vi "FdxCmdTxSAPCreatePortCvi.vi"(8 "error in":errorcluster, 9 "SapCreateIn":T1, 11 "InstrumentHandle":u32) -> (0 "error out":errorcluster, 1 "UdpHandle":u32, 3 "InstrumentHandle":u32)   [LabVIEW 2020, in "AIM664LV.lvlib"]
doc: "Creates an SAP type UDP port to transmit data from a specified UDP connectionless port. Default settings after creation of SAP port are:\n- UDP port enabled\n- Error injection: OFF\n- Skew (redundand mode only): 0 usec.\nTo change settings of the SAP port the function AiFdxCmdTxUDPControl can be used. This function can be used only, if transmitter is not running."
uses:
  AIM664LV.lvlib
  AFDX_LibraryAdmin/FdxGlobalDllPath.vi
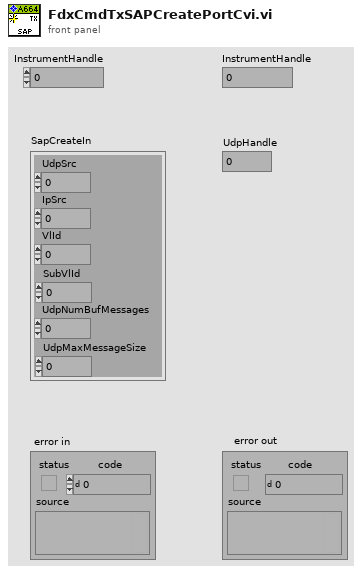
[diagram p1: front panel]
types:
  T1 = cluster{"UdpSrc":u32, "IpSrc":u32, "VlId":u32, "SubVlId":u32, "UdpNumBufMessages":u32, "UdpMaxMessageSize":u32}
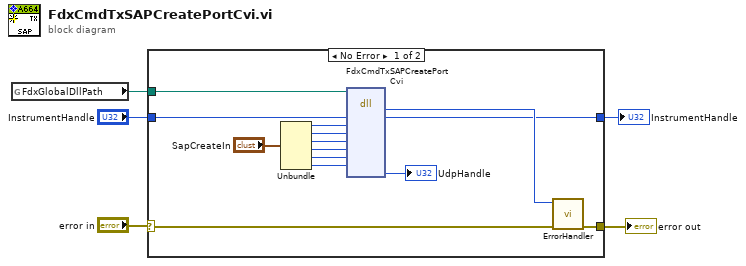
[diagram p0: block diagram]
diagram:
  n1 = global read "FdxGlobalDllPath.vi" "FdxGlobalDllPath"() -> (w3:path)
  n2 = case shown="No Error" "error in" {
    selector: "error in" -> [w18 w21]
    tunnel: [w19 w21] -> w5
    tunnel: w3 -> [w8 _]
    tunnel: "InstrumentHandle" -> [w7 w20]
    tunnel: [w6 w20] -> w1
    frame No Error {
      n3 = Unbundle("SapCreateIn") -> ("UdpSrc"=w14:u32, "IpSrc"=w13:u32, "VlId"=w12:u32, "SubVlId"=w11:u32, "UdpNumBufMessages"=w10:u32, "UdpMaxMessageSize"=w9:u32)
      n4 = dll-call lib="aim_fdx.19.dll" fn="FdxCmdTxSAPCreatePortCvi"(path in=w8, "InstrumentHandle"=w7, "UdpSrc"=w14, "IpSrc"=w13, "VlId"=w12, "SubVlId"=w11, "UdpNumBufMessages"=w10, "UdpMaxMessageSize"=w9) -> ("status"=w17:i32, "InstrumentHandle"=w6:u32, "UdpHandle"=→"UdpHandle":u32)  [unwired: 8 in, 3 out]
      n5 = call "ErrorHandler.vi"("error in"=w18, "AIM Error"=w17) -> ("error out"=w19:errorcluster)  [unwired: 9 in]
    }
    frame Error {
    }
  }
  "error out" <- w5
  "InstrumentHandle" <- w1
